vi "Set Mock as Parent.vi"(8 "error in (no error)":errorcluster, 11 "Mock Class Generator in":refnum<class "Mock Class Generator.lvclass">) -> (0 "error out":errorcluster, 3 "Mock Class Generator out":refnum<class "Mock Class Generator.lvclass">)   [LabVIEW 2020, in "Mock Class Generator.lvclass"]
uses:
  Mock Class Generator.lvclass
  Mock Class Generator.lvclass/Mock Class Generator.ctl
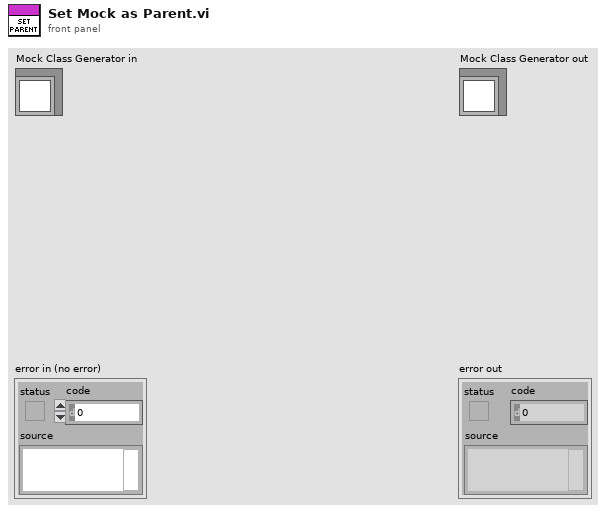
[diagram p1: front panel]
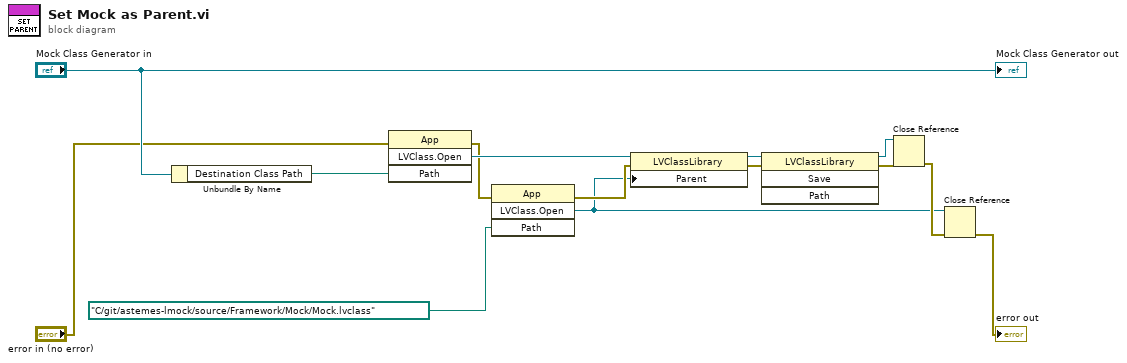
[diagram p0: block diagram]
diagram:
  n1 = Unbundle By Name("Mock Class Generator in") -> ("Destination Class Path"=w12:path)
  n2 = invoke class="App" method="LVClass.Open"(error in="error in (no error)", "Path"=w12) -> (error out=w7:errorcluster, "LVClass.Open"=w11:refnum<vi>)  [unwired: 2 in, 2 out]
  n3 = invoke class="App" method="LVClass.Open"(error in=w7, "Path"=path "C:/git/astemes-lmock/source/Framework/Mock/Mock.lvclass" ("class path")) -> (error out=w14:errorcluster, "LVClass.Open"=w8:refnum<vi>)  [unwired: 2 in, 2 out]
  n4 = property class="LVClassLibrary"(reference=w11, error in=w14, "Parent"=w8) -> (reference out=w3:refnum<vi>, error out=w10:errorcluster)
  n5 = invoke class="LVClassLibrary" method="Save"(reference=w3, error in=w10) -> (reference out=w2:refnum<vi>, error out=w4:errorcluster)  [unwired: 2 in, 2 out]
  n6 = Close Reference(reference=w2, error in (no error)=w4) -> (error out=w9:errorcluster)
  n7 = Close Reference(reference=w8, error in (no error)=w9) -> (error out=→"error out":errorcluster)
  "Mock Class Generator out" <- "Mock Class Generator in"
